vi "SetValveMIXGUIFormat.vi"(10 "State":bool=TRUE, 11 "ValveID":u16(ring) items=["A1", "A2", "A3", "A4", "B1", "B2", "B3", "B4", "B5", "B6", "B7", "B8", "A5", "A6", "A7", "A8"]) -> ()   [LabVIEW 2016]
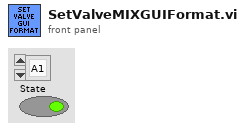
[diagram p1: front panel]
types:
  T1 = enum16{"Release", "Create", "Send", "Wait", "Cancel"}
  T2 = cluster{enum16{"A", "B", "C"}[], enum16{"1", "2", "3", "4", "5", "6", "7", "8"}[], bool[]}
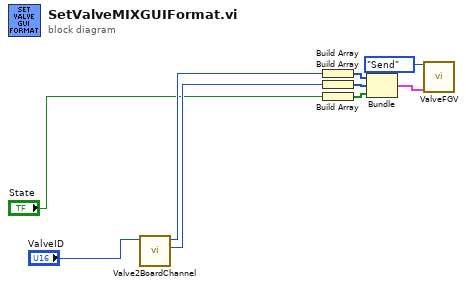
[diagram p0: block diagram]
diagram:
  n1 = call "Valve2BoardChannel.vi"("ValveID"="ValveID") -> ("Channel"=w2:enum16{"1", "2", "3", "4", "5", "6", "7", "8"}, "Flowboard"=w3:enum16{"A", "B", "C"})  [unwired: 9 in]
  n2 = Build Array(w3) -> (w8:enum16{"A", "B", "C"}[])
  n3 = Build Array(w2) -> (w7:enum16{"1", "2", "3", "4", "5", "6", "7", "8"}[])
  n4 = Build Array("State") -> (w6:bool[])
  n5 = Bundle(w8, w7, w6) -> (w5:T2)  [unwired: 1 in]
  n6 = call "ValveFGV.vi"("Valve Data"=w5, "Action"=T1."Send") -> ()  [unwired: 5 in, 5 out]
